vi "V&V Tx Rx.vi"(0 "Configuration Parameters":T1={"Baud"=115200, "Character Length"=8, "Stop Bits"=enum."1.0", "Parity"=enum."None", "Character Spacing (ticks)"=0}, 11 "error in":errorcluster) -> (4 "Number of Read Errors":i32, 6 "Number of Reads Executed":i32, 15 "error out":errorcluster)   [LabVIEW 2012, in "UART_Host_Driver.lvlib" / "UART Driver.lvclass"]
doc: "This example calls the UART Initialize, UART Configure Port, UART Execute Command, and a UART Close."
uses:
  UART Driver.lvclass
  Typedefs/Configuration Parameters.ctl
  FPGA/UART/StopBits.ctl
  FPGA/UART/Parity.ctl
  <vilib>/Instr/_visa.llb/VISA Configure Serial Port (Instr).vi
  FPGA/UART/UART_Firmware.lvlib
  UART_Host_Driver.lvlib
panel:
  out "% Error Rate":dbl
  out "Receive Data":string
  out "Visa Rx Data":string
  in  "stop":bool
  in  "Tx Data":string="ªªªªªªªªªªªªªªªªªªªªªªªªªªªªªªªªªªªªªªªªªªªªªªªªªªªªªªªªªªªªªªªªªªªªªªªªªªªªªªªªªªªªªªªªªªªªªªªªªªªªªªªªªªªªªªªªªªªªªªªªªªªªªªªªªªªªªªªªªªªªªªªªªªªªªªªªªªªªªªªªªªªªªªªªªªªªªªªªªªªªªªªªªªªªªªªªªªªªªªªªªªªªªªªªªªªªªªªªªªªªªªªªªªªªªªªªªªªªªªªªªªªªªªªªªªªªªªªªªªªªªªªªªªªªªªªªªªªªªªªªªªªªªªªªªªªªªªªªªªªªªªªªªªªªªªªªªªªªªªªªªªªªªªªªªªªªªªªªªªªªªªªªªªªªªªªªªªªªªªªªªªªªªªªªªªªªªªªªªªªªªªªªªªªªªªªªªªªªªªªªªªªªªªªªªªªªªªªªªªªªªªªªªªªªªªªªªªªªªªªªªªªªªªªªªªªªªªªªªªªªªªªªªªªªªªªªªªªªªªªªªªªªªªªªªªªªªªªªªªªª"
  # "500 bytes"
  # "AAAA AAAA AAAA AAAA AAAA AAAA AAAA AAAA AAAA AAAA AAAA AAAA AAAA AAAA AAAA AAAA AAAA AAAA AAAA AAAA AAAA AAAA AAAA AAAA AAAA AAAA AAAA AAAA AAAA AAAA AAAA AAAA AAAA AAAA AAAA AAAA AAAA AAAA AAAA AAAA AAAA AAAA AAAA AAAA AAAA AAAA AAAA AAAA AAAA AAAA AAAA AAAA AAAA AAAA AAAA AAAA AAAA AAAA AAAA AAAA AAAA AAAA AAAA AAAA AAAA AAAA AAAA AAAA AAAA AAAA AAAA AAAA AAAA AAAA AAAA AAAA AAAA AAAA AAAA AAAA AAAA AAAA AAAA AAAA AAAA AAAA AAAA AAAA AAAA AAAA AAAA AAAA AAAA AAAA AAAA AAAA AAAA AAAA AAAA AAAA AAAA AAAA AAAA AAAA AAAA AAAA AAAA AAAA AAAA AAAA AAAA AAAA AAAA AAAA AAAA AAAA AAAA AAAA AAAA AAAA AAAA AAAA AAAA AAAA AAAA AAAA AAAA AAAA AAAA AAAA AAAA AAAA AAAA AAAA AAAA AAAA AAAA AAAA AAAA AAAA AAAA AAAA AAAA AAAA AAAA AAAA AAAA AAAA AAAA AAAA AAAA AAAA AAAA AAAA AAAA AAAA AAAA AAAA AAAA AAAA AAAA AAAA AAAA AAAA AAAA AAAA AAAA AAAA AAAA AAAA AAAA AAAA AAAA AAAA AAAA AAAA AAAA AAAA AAAA AAAA AAAA AAAA AAAA AAAA AAAA AAAA AAAA AAAA AAAA AAAA AAAA AAAA AAAA AAAA AAAA AAAA AAAA AAAA AAAA AAAA AAAA AAAA AAAA AAAA AAAA AAAA AAAA AAAA AAAA AAAA AAAA AAAA AAAA AAAA AAAA AAAA AAAA AAAA AAAA AAAA AAAA AAAA AAAA AAAA AAAA AAAA AAAA AAAA AAAA AAAA AAAA AAAA AAAA AAAA AAAA AAAA AAAA AAAA AAAA AAAA AAAA AAAA AAAA AAAA AAAA AAAA AAAA AAAA AAAA AAAA"
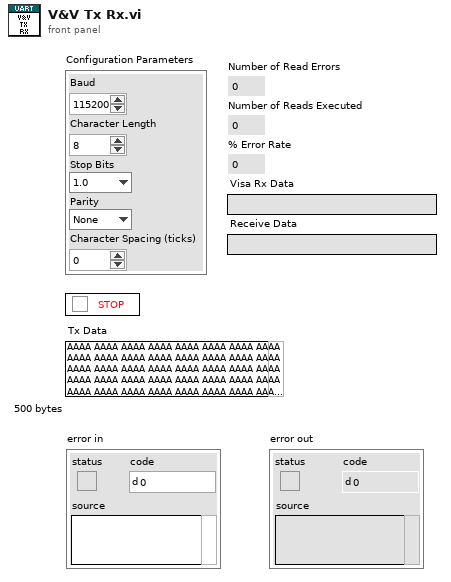
[diagram p1: front panel]
types:
  T1 = typedef "UART_Host_Driver.lvlib/Configuration Parameters.ctl" = cluster{"Baud":u32, "Character Length":u8, "Stop Bits":T2, "Parity":T3, "Character Spacing (ticks)":u32}
  T2 = typedef "UART_Firmware.lvlib/StopBits.ctl" = enum8{"1.0", "1.5", "2.0"}
  T3 = typedef "UART_Firmware.lvlib/Parity.ctl" = enum8{"None", "Even", "Odd"}
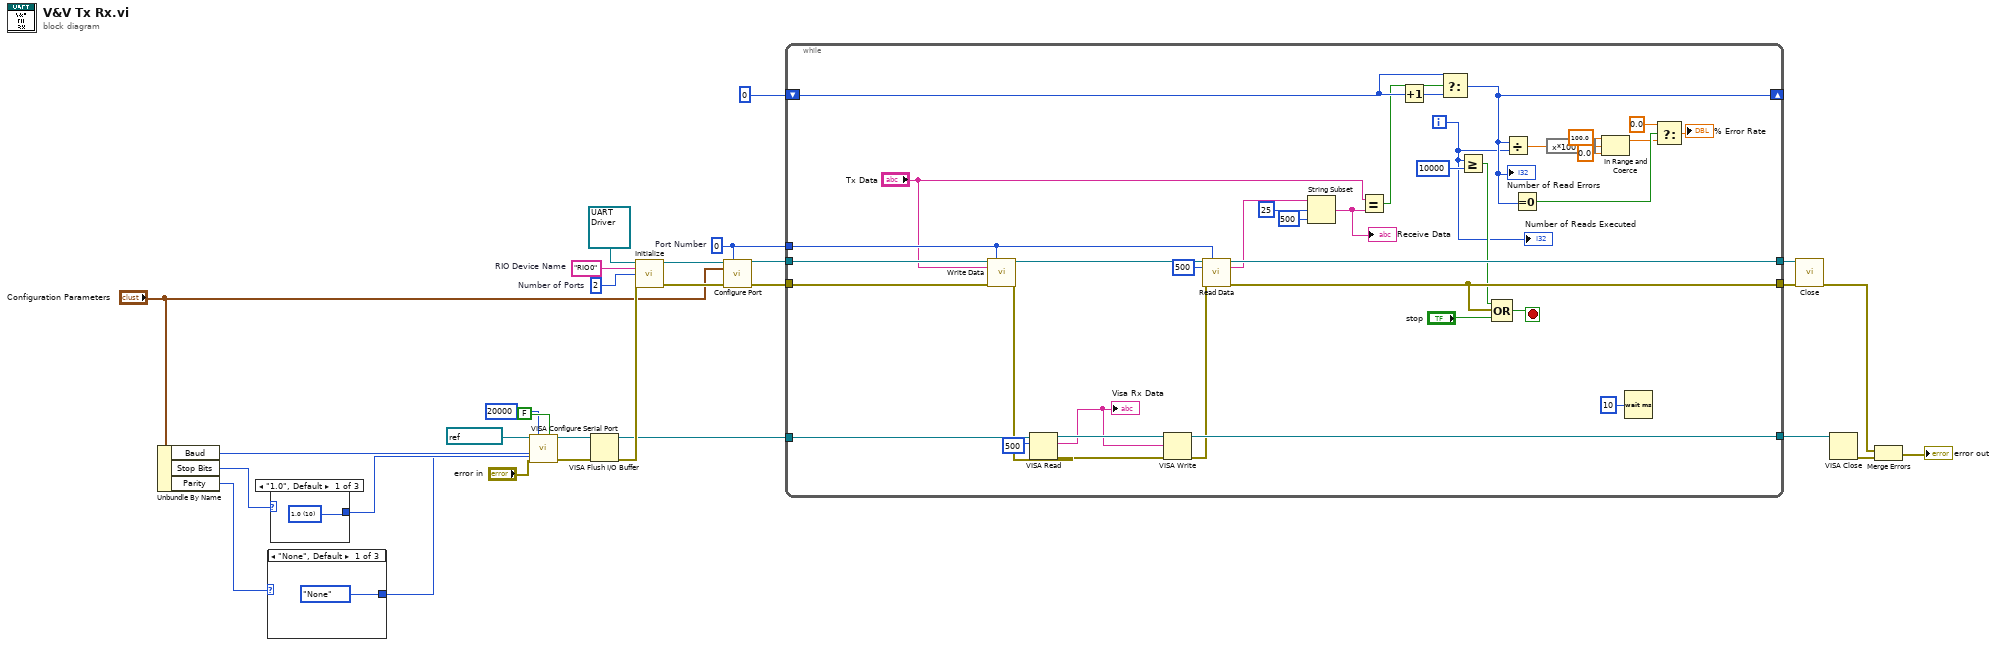
[diagram p0: block diagram]
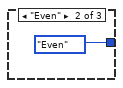
[diagram p2: hidden frame]
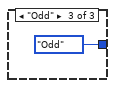
[diagram p3: hidden frame]
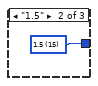
[diagram p4: hidden frame]
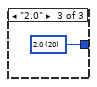
[diagram p5: hidden frame]
diagram:
  w22 = u8 0  # Port Number
  w25 = u8 2  # Number of Ports
  w26 = "RIO0"  # RIO Device Name
  n1 = Unbundle By Name("Configuration Parameters") -> ("Baud"=w8:u32, "Stop Bits"=w7:T2, "Parity"=w5:T3)
  n2 = case shown="\"None\", Default" w5 {
    tunnel: [enum16{"None", "Odd", "Even", "Mark", "Space"}."None" ("parity (0:none)") enum16{"None", "Odd", "Even", "Mark", "Space"}."Even" ("parity (0:none)") enum16{"None", "Odd", "Even", "Mark", "Space"}."Odd" ("parity (0:none)")] -> w4
    frame "None", Default {
    }
    frame "Even" {
    }
    frame "Odd" {
    }
  }
  n3 = case shown="\"1.0\", Default" w7 {
    tunnel: [w33 w34 w35] -> w6
    frame "1.0", Default {
      w33 = u16 10 items=["1.0"=10, "1.5"=15, "2.0"=20] ("stop bits (10: 1 bit)")
    }
    frame "1.5" {
      w34 = u16 15 items=["1.0"=10, "1.5"=15, "2.0"=20] ("stop bits (10: 1 bit)")
    }
    frame "2.0" {
      w35 = u16 20 items=["1.0"=10, "1.5"=15, "2.0"=20] ("stop bits (10: 1 bit)")
    }
  }
  n4 = call-poly "VISA Configure Serial Port"("VISA resource name"=refnum<visa-resource-name> "COM1", "timeout (10sec)"=u32 20000, "Enable Termination\nChar (T)"=FALSE ("Enable Termination\nChar (T)"), "baud rate (9600)"=w8, "parity (0:none)"=w4, "error in (no error)"="error in", "stop bits (10: 1 bit)"=w6) -> ("VISA resource name out"=w16:refnum<visa-resource-name>, "error out"=w17:errorcluster)  [unwired: 7 in]
  n5 = VISA Flush I/O Buffer(VISA resource name=w16, error in (no error)=w17) -> (VISA resource name out=w12:refnum<visa-resource-name>, error out=w15:errorcluster)  [unwired: 1 in]
  n6 = call-dynamic "Initialize.vi"("UART Driver in"=refnum<class "UART Driver.lvclass"> refnum, "RIO Device Name"=w26, "Number of UART Controllers"=w25, "error in"=w15) -> ("UART Driver out"=w29:refnum<class "UART Driver.lvclass">, "error out"=w28:errorcluster)  [unwired: 10 in]
  n7 = call-dynamic "Configure Port.vi"("UART Driver in"=w29, "Controller Number"=w22, "Configuration Parameters"="Configuration Parameters", "error in"=w28) -> ("UART Driver out"=w24:refnum<class "UART Driver.lvclass">, "error out"=w23:errorcluster)  [unwired: 10 in]
  n8 = while {
    tunnel: w24 -> [w73]
    tunnel: w23 -> [w72]
    tunnel: w22 -> [w57]
    tunnel: [w52] -> w21
    tunnel: [w58] -> w20
    tunnel: w12 -> [w69]
    shift-right: [w37] -> _
    shift-left: 0 -> [w66]
    tunnel: [w62] -> w13
    i -> [w36]
    stop <- w51 stop-if-true
    n9 = call-dynamic "Write Data.vi"("UART Driver in"=w73, "Port Number"=w57, "Tx Data"="Tx Data", "error in"=w72) -> ("UART Driver out"=w60:refnum<class "UART Driver.lvclass">, "error out"=w68:errorcluster)  [unwired: 10 in]
    n10 = VISA Read(VISA resource name=w69, byte count=u32 500, error in (no error)=w68) -> (VISA resource name out=w65:refnum<visa-resource-name>, read buffer=w63:string, error out=w64:errorcluster)  [unwired: 1 out]
    "Visa Rx Data" <- w63
    n11 = VISA Write(VISA resource name=w65, write buffer=w63, error in (no error)=w64) -> (VISA resource name out=w62:refnum<visa-resource-name>, error out=w59:errorcluster)  [unwired: 1 out]
    n12 = call-dynamic "Read Data.vi"("UART Driver in"=w60, "Port Number"=w57, "Rx byte count"=u32 500, "error in"=w59) -> ("UART Driver out"=w58:refnum<class "UART Driver.lvclass">, "Receive Data"=w54:string, "error out"=w52:errorcluster)  [unwired: 9 in]
    n13 = String Subset(string=w54, offset (0)=25 ("length (rest)"), length (rest)=500 ("length (rest)")) -> (substring=w47:string)
    "Receive Data" <- w47
    n14 = Equal?(x="Tx Data", y=w47) -> (x = y?=w53:bool)
    n15 = Increment(x=w66) -> (x+1=w67:i32)
    n16 = Select(t=w66, s=w53, f=w67) -> (s? t:f=w37:i32)
    "Number of Read Errors" <- w37
    n17 = Greater Or Equal?(x=w36, y=10000) -> (x >= y?=w40:bool)
    n18 = Compound Arithmetic op=OR(w40, w52, "stop") -> (w51:bool)
    n19 = Divide(x=w37, y=w36) -> (x/y=w46:dbl)
    n20 = Equal To 0?(x=w37) -> (x = 0?=w45:bool)
    n21 = expression code="x*100"(w46) -> (w39:dbl)
    n22 = In Range and Coerce(upper limit=100.0, x=w39, lower limit=0.0) -> (coerced(x)=w42:dbl)  [unwired: 1 out]
    n23 = Wait (ms)(milliseconds to wait=u32 10) -> ()  [unwired: 1 out]
    n24 = Select(t=0.0, s=w45, f=w42) -> (s? t:f=→"% Error Rate":dbl)
    "Number of Reads Executed" <- w36
  }
  n25 = call-dynamic "Close.vi"("UART Driver in"=w20, "error in"=w21) -> ("error out"=w10:errorcluster)  [unwired: 13 in]
  n26 = VISA Close(VISA resource name=w13) -> (error out=w11:errorcluster)  [unwired: 1 in]
  n27 = Merge Errors(w10, w11) -> (→"error out":errorcluster)
